vi "Untitled 1.vi"() -> ()   [LabVIEW 2009]
uses:
  <vilib>/vision/Image Controls.llb/IMAQ Image.ctl
  <vilib>/Analysis/3filter.llb/Filter Passband Type.ctl
  <vilib>/Analysis/3filter.llb/Butterworth Filter (DBL).vi
  <vilib>/vision/NI_Vision_Development_Module.lvlib
  <vilib>/Analysis/NI_AALBase.lvlib
panel:
  in  "playtime":dbl=1.0
  out "Numeric 2":i32
  in  "Numeric":i32=1250
  out "Boolean":bool
  in  "low cutoff freq: fl":dbl=0.12500000000000006 format="%0.4f"
  out "Waveform Graph":dbl[](graph)
  in  "high cutoff freq: fh":dbl=0.45000000000000007 format="%0.2f"
  in  "sampling freq: fs":dbl=1.0 format="%0.2f"
  out "ROI Pixel Statistics":T1
  out "Image Out 2":T2
  out "Line Profile  BLUE":cluster{"x0":sgl, "dx":sgl, "Pixels Line":sgl[]}(graph) caption="Line Profile"
  out "Line Profile RED":cluster{"x0":sgl, "dx":sgl, "Pixels Line":sgl[]}(graph) caption="Line Profile"
  out "Image Out":T2
  out "Image 2":T2(plugin-control)
  out "Image":T2(plugin-control)
  in  "stop":bool
  in  "AVI Path":path
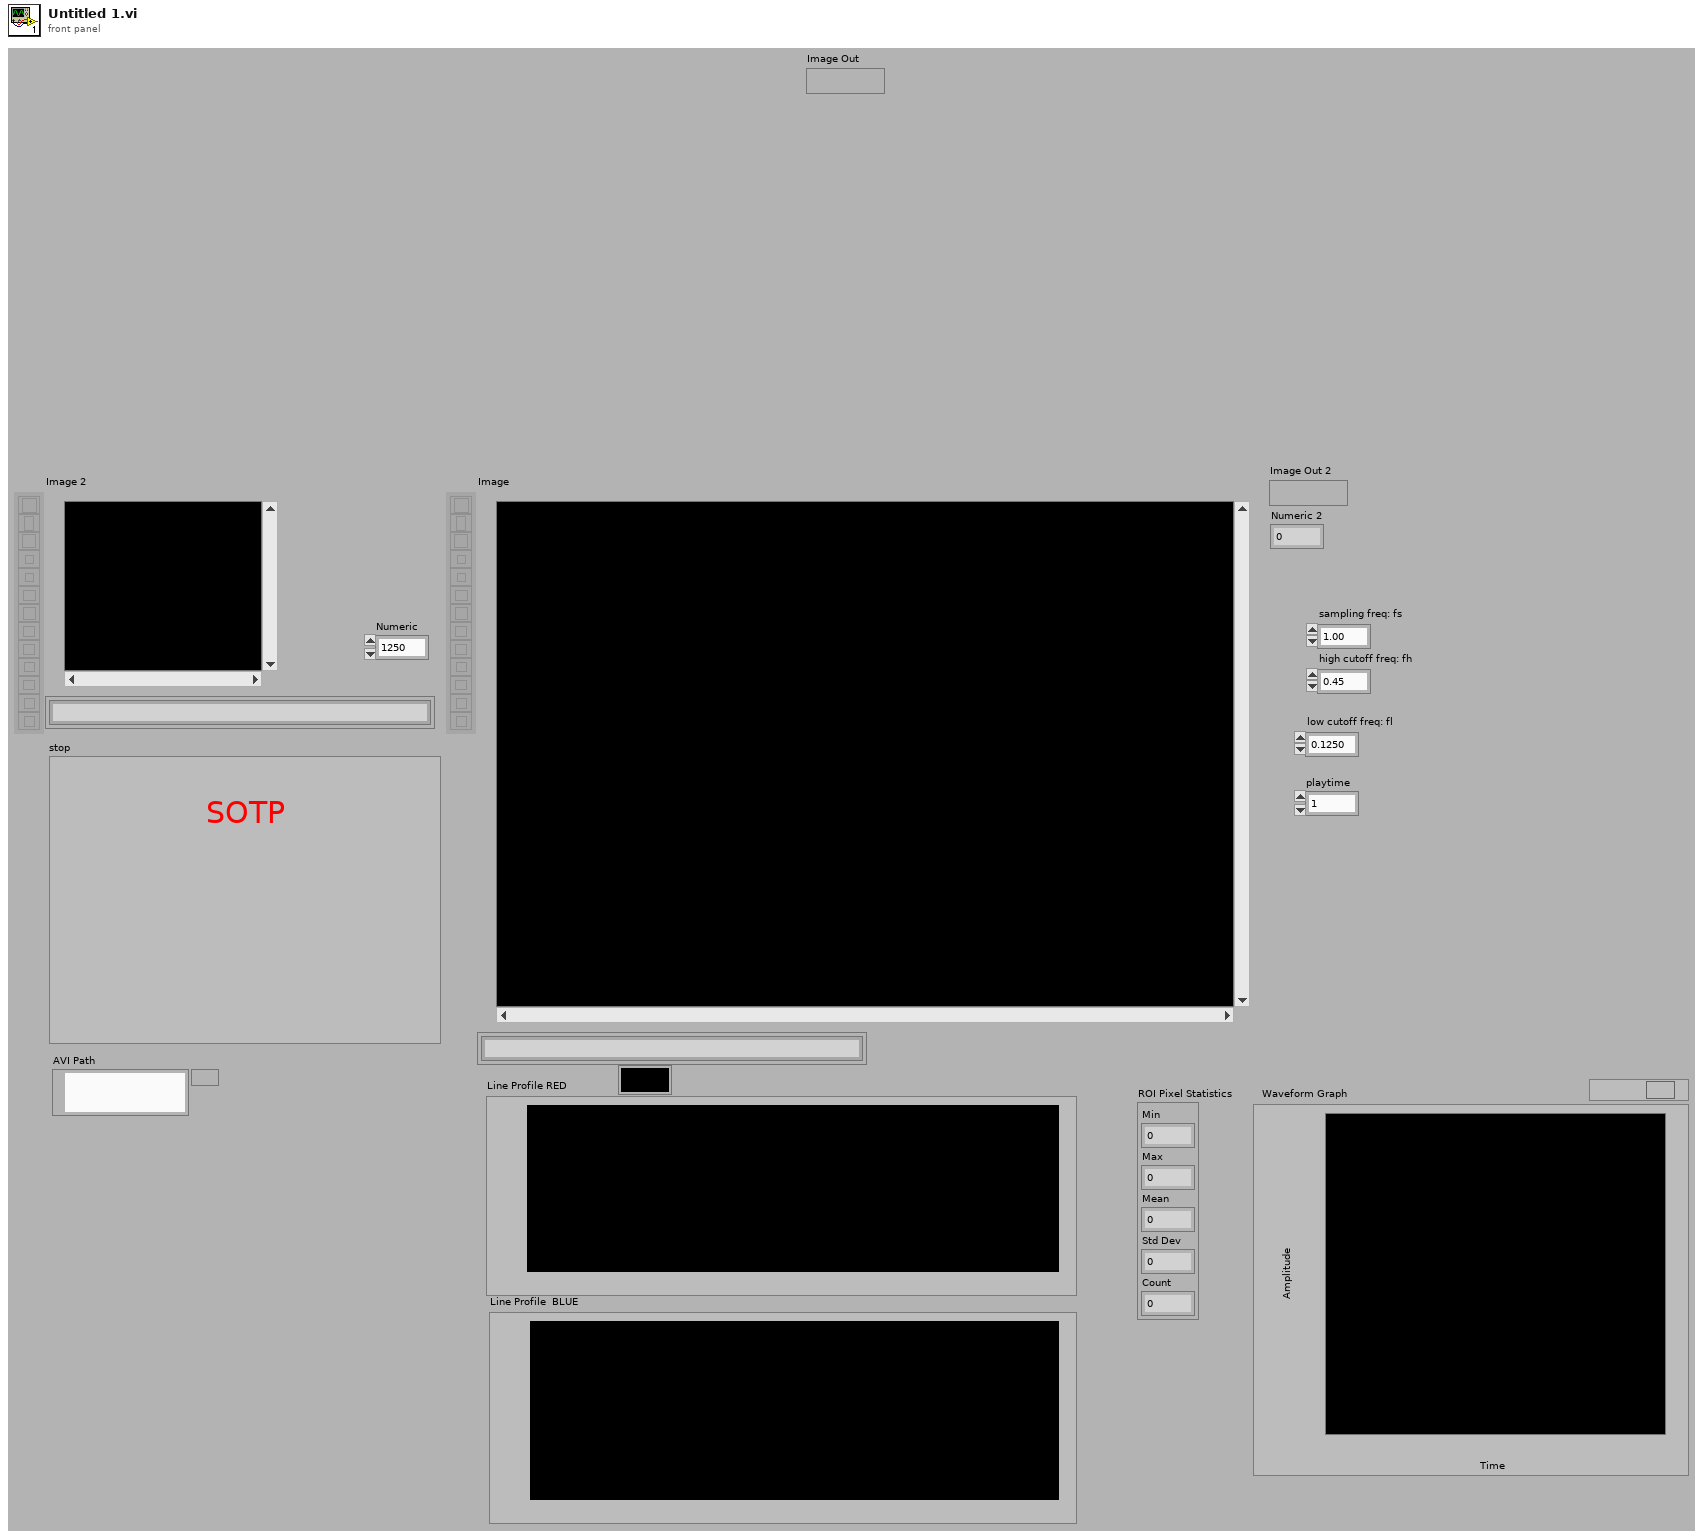
[diagram p1: front panel]
types:
  T1 = cluster{"Min":sgl, "Max":sgl, "Mean":sgl, "Std Dev":sgl, "Count":i32}
  T2 = typedef "IMAQ Image.ctl" = refnum<image>
  T3 = typedef "NI_AALBase.lvlib/Filter Passband Type.ctl" = enum32{"Lowpass", "Highpass", "Bandpass", "Bandstop"}
  T4 = cluster{"Left":i32, "Top":i32, "Right":i32, "Bottom":i32}
  T5 = cluster{"Global Rectangle":i32[], "Contours":cluster{"ID":enum32{"External", "Internal"}, "Type":u32, "Coordinates":i32[]}[]}
  T6 = cluster{"ID":enum32{"External", "Internal"}, "Type":u32, "Coordinates":i32[]}[]
  T7 = cluster{"ID":enum32{"External", "Internal"}, "Type":u32, "Coordinates":i32[]}
  T8 = typedef "AviRefnum.ctl" = refnum<k1>
  T9 = typedef "Image Type" = u32
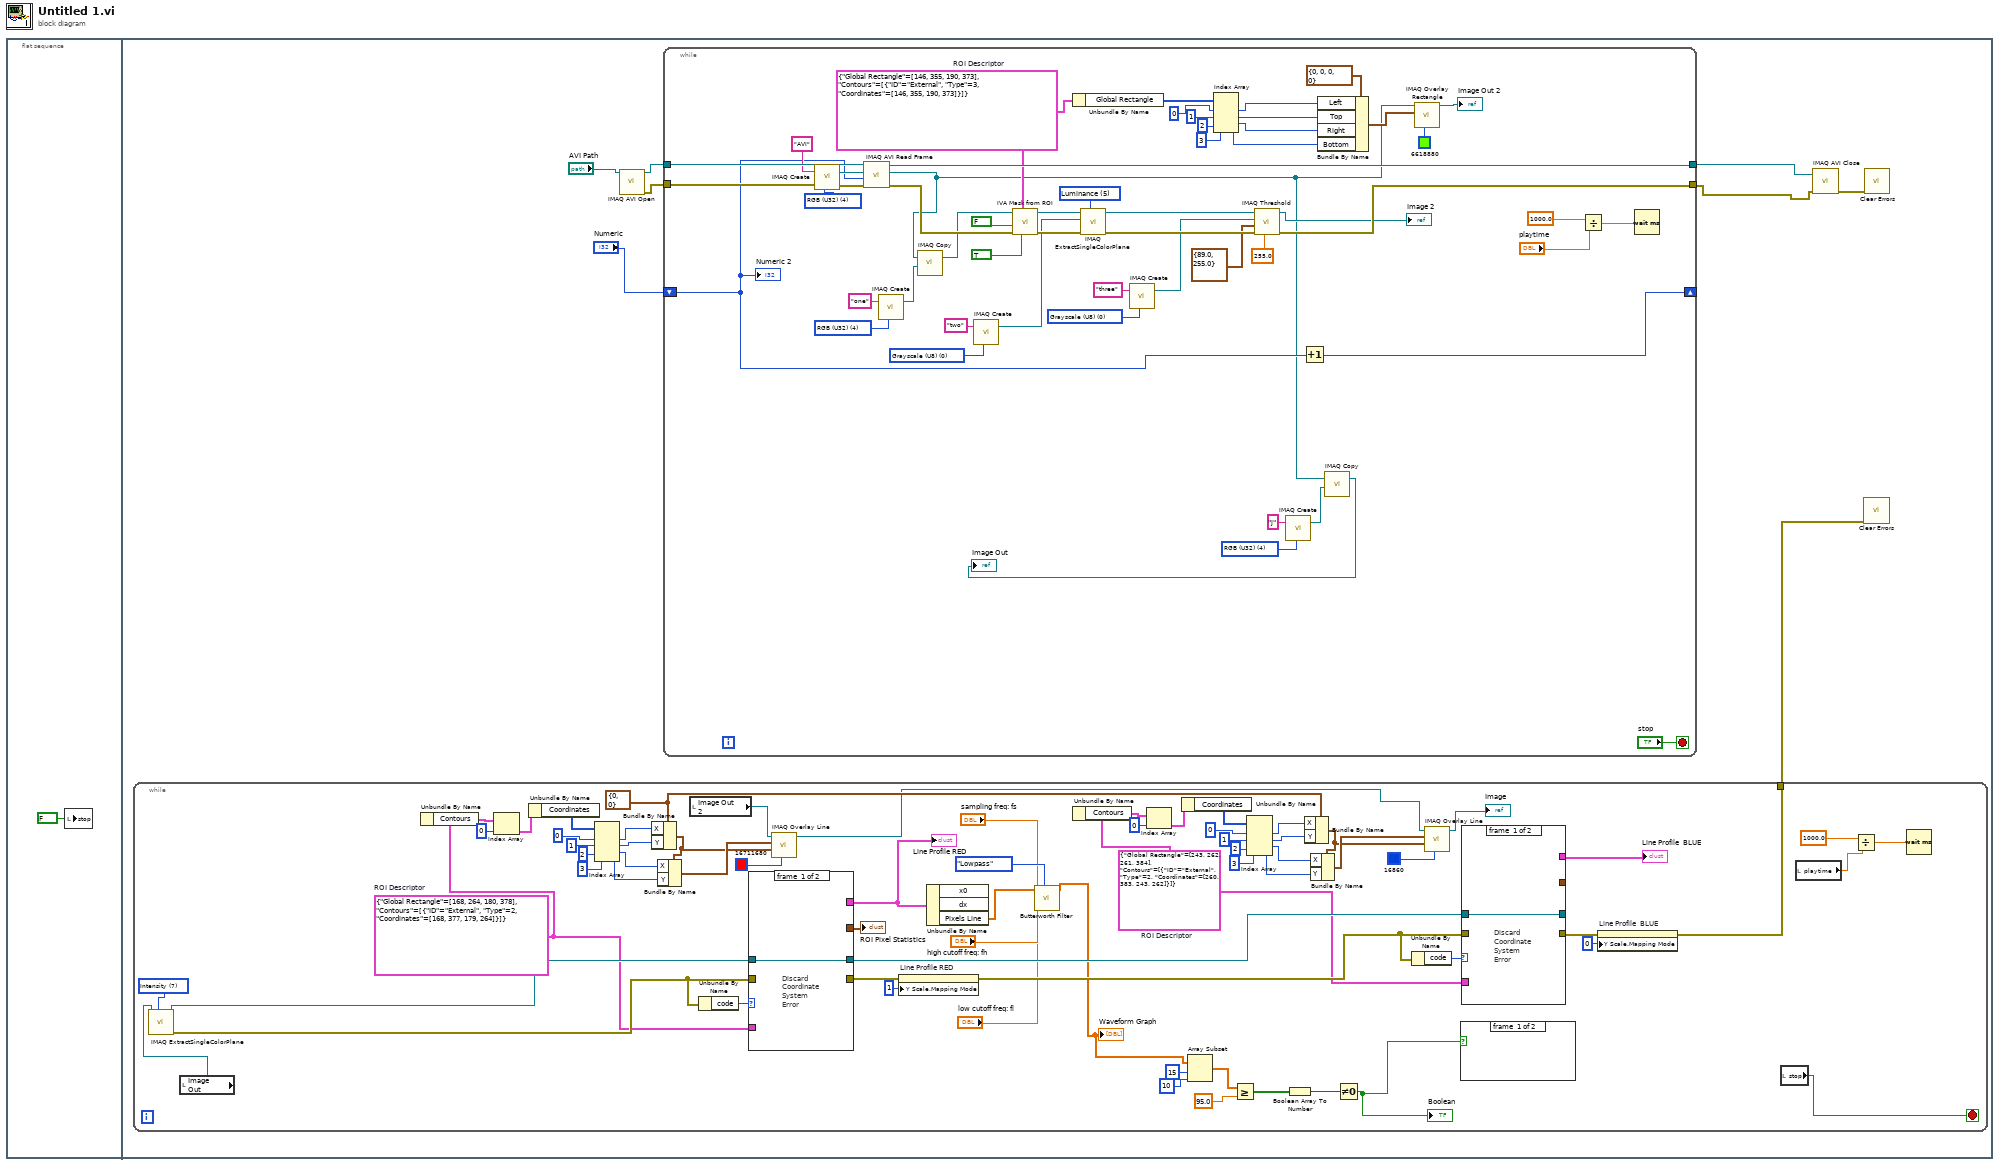
[diagram p0: block diagram]
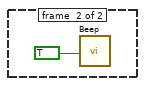
[diagram p2: hidden frame]
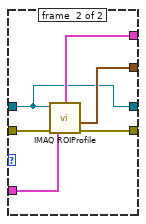
[diagram p3: hidden frame]
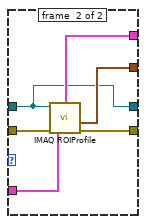
[diagram p4: hidden frame]
diagram:
  n1 = flat-sequence {
    frame #0 {
      n2 = local write "stop"(FALSE ("stop")) -> ()
    }
    frame #1 {
      n3 = while {
        tunnel: [w64] -> w2
        stop <- w65 stop-if-true
        w32 = cluster{"X":i32, "Y":i32} {"X"=0, "Y"=0} ("End Point")
        w35 = T5 {"Global Rectangle"=[243, 262, 261, 384], "Contours"=[{"ID"=enum."External", "Type"=2, "Coordinates"=[260, 383, 243, 262]}]}  # ROI Descriptor
        w55 = T5 {"Global Rectangle"=[168, 264, 180, 378], "Contours"=[{"ID"=enum."External", "Type"=2, "Coordinates"=[168, 377, 179, 264]}]}  # ROI Descriptor
        w78 = 7 items=["Red", "Green", "Blue", "Hue", "Saturation", "Luminance", "Value", "Intensity"] ("Color Plane")
        n4 = local read "Image Out"() -> (w66:T2)
        n5 = call "IMAQ ExtractSingleColorPlane"("Color Plane"=w78, "Image Src"=w66) -> ("error out"=w77:errorcluster, "Image Dst Out"=w73:T2)  [unwired: 2 in, 6 out]
        n6 = Unbundle By Name(w55) -> ("Contours"=w52:T6)
        n7 = Index Array(array=w52, index=0) -> (element=w50:T7)
        n8 = Unbundle By Name(w50) -> ("Coordinates"=w49:i32[])
        n9 = Index Array(array=w49, index #1=0 ("index"), index #2=1 ("index"), index #3=2 ("index"), index #4=3 ("index")) -> (element #1=w59:i32, element #2=w58:i32, element #3=w57:i32, element #4=w56:i32)
        n10 = Bundle By Name(cluster=w32, "X"=w59, "Y"=w58) -> (w33:cluster{"X":i32, "Y":i32})
        n11 = Bundle By Name(cluster=w33, "X"=w57, "Y"=w56) -> (w34:cluster{"X":i32, "Y":i32})
        n12 = local read "Image Out 2"() -> (w54:T2)
        n13 = Unbundle By Name(w77) -> ("code"=w72:i32)
        n14 = case shown="Default" w72 {
          tunnel: w77 -> [_ w93]
          tunnel: [_ w92] -> w27
          tunnel: [_ w91] -> w75
          tunnel: w73 -> [w87 w88]
          tunnel: [_ w90] -> w25
          tunnel: w55 -> [_ w89]
          tunnel: [w87 w88] -> w69
          frame #0 {
            # "Discard\nCoordinate\nSystem\nError"
          }
          frame #1 {
            n15 = call "IMAQ ROIProfile"("error in (no error)"=w93, "ROI Descriptor"=w89, "Image"=w88) -> ("ROI Pixel Statistics"=w92:T1, "error out"=w91:errorcluster, "ROI Graph"=w90:cluster{"x0":sgl, "dx":sgl, "Pixels Line":sgl[]})  [unwired: 3 out]
          }
        }
        "Line Profile RED" <- w25
        "ROI Pixel Statistics" <- w27
        n16 = call "IMAQ Overlay Line"("Color"=u32 16711680, "End Point"=w33, "Start Point"=w34, "Image"=w54) -> ("Image Out"=w29:T2)  [unwired: 6 in, 1 out]
        n17 = property on="Line Profile RED" class="WFGraph"(error in=w75, "Y Scale.Mapping Mode"=u8 1) -> (error out=w74:errorcluster)  [unwired: 1 in, 1 out]
        n18 = Unbundle By Name(w25) -> ("Pixels Line"=w24:sgl[])  [unwired: 2 out]
        n19 = call-poly <vilib>:"Butterworth Filter.vi"("filter type"=Filter_Passband_Type."Lowpass", "low cutoff freq: fl"="low cutoff freq: fl", "high cutoff freq: fh"="high cutoff freq: fh", "sampling freq: fs"="sampling freq: fs", "X"=w24) -> ("Filtered X"=w20:dbl[])  [unwired: 3 in, 1 out]
        "Waveform Graph" <- w20
        n20 = Unbundle By Name(w35) -> ("Contours"=w45:T6)
        n21 = Index Array(array=w45, index=0) -> (element=w47:T7)
        n22 = Unbundle By Name(w47) -> ("Coordinates"=w48:i32[])
        n23 = Array Subset(array=w20, index=15, length=10) -> (w17:dbl[])
        n24 = Greater Or Equal?(x=w17, y=95.0) -> (x >= y?=w15:bool[])
        n25 = Index Array(array=w48, index #1=0 ("index"), index #2=1 ("index"), index #3=2 ("index"), index #4=3 ("index")) -> (element #1=w40:i32, element #2=w41:i32, element #3=w42:i32, element #4=w43:i32)
        n26 = Boolean Array To Number(Boolean array=w15) -> (number=w12:u32)
        n27 = Bundle By Name(cluster=w32, "X"=w40, "Y"=w41) -> (w30:cluster{"X":i32, "Y":i32})
        n28 = Bundle By Name(cluster=w30, "X"=w42, "Y"=w43) -> (w31:cluster{"X":i32, "Y":i32})
        n29 = Not Equal To 0?(x=w12) -> (x != 0?=w10:bool)
        "Boolean" <- w10
        n30 = Unbundle By Name(w74) -> ("code"=w67:i32)
        n31 = call "IMAQ Overlay Line"("Color"=u32 16860, "End Point"=w30, "Start Point"=w31, "Image"=w29) -> ("Image Out"=→"Image":T2)  [unwired: 6 in, 1 out]
        n32 = case shown="True" w10 {
          frame #0 {
          }
          frame #1 {
            n33 = call <vilib>:"Beep.vi"("use system alert? (T)"=TRUE) -> ()  [unwired: 11 in]
          }
        }
        n34 = case shown="Default" w67 {
          tunnel: w74 -> [_ w86]
          tunnel: [_ w85] -> _
          tunnel: [_ w84] -> w70
          tunnel: w69 -> [w80 w81]
          tunnel: [_ w83] -> w68
          tunnel: w35 -> [_ w82]
          tunnel: [w80 w81] -> _
          frame #0 {
            # "Discard\nCoordinate\nSystem\nError"
          }
          frame #1 {
            n35 = call "IMAQ ROIProfile"("error in (no error)"=w86, "ROI Descriptor"=w82, "Image"=w81) -> ("ROI Pixel Statistics"=w85:T1, "error out"=w84:errorcluster, "ROI Graph"=w83:cluster{"x0":sgl, "dx":sgl, "Pixels Line":sgl[]})  [unwired: 3 out]
          }
        }
        "Line Profile  BLUE" <- w68
        n36 = property on="Line Profile  BLUE" class="WFGraph"(error in=w70, "Y Scale.Mapping Mode"=u8 0) -> (error out=w64:errorcluster)  [unwired: 1 in, 1 out]
        n37 = local read "stop"() -> (w65:bool)
        n38 = local read "playtime"() -> (w11:dbl)
        n39 = Divide(x=1000.0, y=w11) -> (x/y=w14:dbl)
        n40 = Wait (ms)(milliseconds to wait=w14) -> ()  [unwired: 1 out]
      }
      n41 = call "IMAQ AVI Open"("AVI Path"="AVI Path") -> ("error out"=w4:errorcluster, "Avi Refnum"=w5:T8)  [unwired: 9 in]
      n42 = while {
        tunnel: w5 -> [w144]
        tunnel: w4 -> [w147]
        tunnel: [w135] -> w6
        tunnel: [w141] -> w7
        shift-right: [w130] -> _
        shift-left: "Numeric" -> [w129]
        stop <- "stop" stop-if-true
        w99 = T9 4 items=["Grayscale (U8)", "Grayscale (I16)", "Grayscale (SGL)", "Complex (CSG)", "RGB (U32)", "HSL (U32)", "RGB (U64)", "Grayscale (U16)"] ("Image Type")
        w105 = T9 0 items=["Grayscale (U8)", "Grayscale (I16)", "Grayscale (SGL)", "Complex (CSG)", "RGB (U32)", "HSL (U32)", "RGB (U64)", "Grayscale (U16)"] ("Image Type")
        w111 = 5 items=["Red", "Green", "Blue", "Hue", "Saturation", "Luminance", "Value", "Intensity"] ("Color Plane")
        w131 = T9 0 items=["Grayscale (U8)", "Grayscale (I16)", "Grayscale (SGL)", "Complex (CSG)", "RGB (U32)", "HSL (U32)", "RGB (U64)", "Grayscale (U16)"] ("Image Type")
        w132 = T9 4 items=["Grayscale (U8)", "Grayscale (I16)", "Grayscale (SGL)", "Complex (CSG)", "RGB (U32)", "HSL (U32)", "RGB (U64)", "Grayscale (U16)"] ("Image Type")
        w128 = T5 {"Global Rectangle"=[146, 355, 190, 373], "Contours"=[{"ID"=enum."External", "Type"=3, "Coordinates"=[146, 355, 190, 373]}]}  # ROI Descriptor
        w142 = T9 4 items=["Grayscale (U8)", "Grayscale (I16)", "Grayscale (SGL)", "Complex (CSG)", "RGB (U32)", "HSL (U32)", "RGB (U64)", "Grayscale (U16)"] ("Image Type")
        n43 = call "IMAQ Create"("Image Name"="AVI", "Image Type"=w142, "error in (no error)"=w147) -> ("New Image"=w145:T2, "error out"=w146:errorcluster)  [unwired: 2 in]
        n44 = call "IMAQ AVI Read Frame"("error in (no error)"=w146, "Frame Number"=w129, "Image"=w145, "Avi Refnum"=w144) -> ("error out"=w136:errorcluster, "Image Out"=w96:T2, "Avi Refnum (duplicate)"=w141:T8)  [unwired: 4 in, 1 out]
        n45 = call "IMAQ Create"("Image Name"="one", "Image Type"=w132) -> ("New Image"=w134:T2)  [unwired: 3 in, 1 out]
        n46 = call "IMAQ Copy"("Image Dst"=w134, "Image Src"=w96) -> ("Image Dst Out"=w115:T2)  [unwired: 4 in, 1 out]
        n47 = call "IMAQ Create"("Image Name"="two", "Image Type"=w131) -> ("New Image"=w101:T2)  [unwired: 3 in, 1 out]
        n48 = call <vilib>:"IVA Mask from ROI.vi"("Shrink"=TRUE, "ROI Descriptor"=w128, "error in (no error)"=w136, "Out / In"=FALSE, "Image Src"=w115) -> ("error out"=w113:errorcluster, "Image Out"=w110:T2)  [unwired: 5 out]
        n49 = Unbundle By Name(w128) -> ("Global Rectangle"=w124:i32[])
        n50 = call "IMAQ ExtractSingleColorPlane"("Color Plane"=w111, "error in (no error)"=w113, "Image Dst"=w101, "Image Src"=w110) -> ("error out"=w109:errorcluster, "Image Dst Out"=w107:T2)  [unwired: 6 out]
        n51 = call "IMAQ Create"("Image Name"="three", "Image Type"=w105) -> ("New Image"=w103:T2)  [unwired: 3 in, 1 out]
        n52 = Index Array(array=w124, index #1=0 ("index"), index #2=1 ("index"), index #3=2 ("index"), index #4=3 ("index")) -> (element #1=w123:i32, element #2=w122:i32, element #3=w121:i32, element #4=w120:i32)
        n53 = call "IMAQ Threshold"("Replace Value"=sgl 255.0, "error in (no error)"=w109, "Range"=cluster{"Lower value":sgl, "Upper value":sgl} {"Lower value"=89.0, "Upper value"=255.0}, "Image Dst"=w103, "Image Src"=w107) -> ("error out"=w135:errorcluster, "Image Dst Out"=→"Image 2":T2)  [unwired: 1 in, 4 out]
        n54 = call "IMAQ Create"("Image Name"="j", "Image Type"=w99) -> ("New Image"=w97:T2)  [unwired: 3 in, 1 out]
        n55 = Increment(x=w129) -> (x+1=w130:i32)
        n56 = Bundle By Name(cluster=T4 {"Left"=0, "Top"=0, "Right"=0, "Bottom"=0} ("Rectangle"), "Left"=w123, "Top"=w122, "Right"=w121, "Bottom"=w120) -> (w126:T4)
        n57 = call "IMAQ Copy"("Image Dst"=w97, "Image Src"=w96) -> ("Image Dst Out"=→"Image Out":T2)  [unwired: 4 in, 1 out]
        n58 = call "IMAQ Overlay Rectangle"("Color"=u32 6618880, "Rectangle"=w126, "Image"=w96) -> ("Image Out"=→"Image Out 2":T2)  [unwired: 7 in, 1 out]
        n59 = Divide(x=1000.0, y="playtime") -> (x/y=w139:dbl)
        n60 = Wait (ms)(milliseconds to wait=w139) -> ()  [unwired: 1 out]
        "Numeric 2" <- w129
      }
      n61 = call "IMAQ AVI Close"("error in (no error)"=w6, "Avi Refnum"=w7) -> ("error out"=w8:errorcluster)  [unwired: 9 in]
      n62 = call <vilib>:"Clear Errors.vi"("error in (no error)"=w2) -> ()  [unwired: 6 in, 1 out]
      n63 = call <vilib>:"Clear Errors.vi"("error in (no error)"=w8) -> ()  [unwired: 6 in, 1 out]
    }
  }
